vi "RTS Door Opener Server Side.vi"() -> ()   [LabVIEW 2016]
uses:
  <vilib>/Utility/file.llb/Read Delimited Spreadsheet (string).vi
  Type Definitions/RTS Door Open Close Pattern.ctl
  Type Definitions/RTS Door OpenClose Pattern.ctl
  Type Definitions/RTS Door Action.ctl
panel:
  out "Door Open/Close Pattern 4":T1=[{"Door Action"=enum."OPEN", "Timer (Seconds)"=5}, {"Door Action"=enum."CLOSE", "Timer (Seconds)"=5}, {"Door Action"=enum."DELAY", "Timer (Seconds)"=5}, {"Door Action"=enum."REPEAT", "Timer (Seconds)"=0}]
  out "Door Open/Close Pattern 3":T1=[{"Door Action"=enum."OPEN", "Timer (Seconds)"=5}, {"Door Action"=enum."CLOSE", "Timer (Seconds)"=5}, {"Door Action"=enum."DELAY", "Timer (Seconds)"=5}, {"Door Action"=enum."REPEAT", "Timer (Seconds)"=0}]
  out "Door Open/Close Pattern":T1=[{"Door Action"=enum."OPEN", "Timer (Seconds)"=5}, {"Door Action"=enum."CLOSE", "Timer (Seconds)"=5}, {"Door Action"=enum."DELAY", "Timer (Seconds)"=5}, {"Door Action"=enum."REPEAT", "Timer (Seconds)"=0}]
  in  "OK":bool
  out "Elapsed days":i32
  out "End Time":timestamp format="%<%I:%M:%S%3u %p\n%m/%d/%Y>T"
  out "Start Time":timestamp format="%<%I:%M:%S%3u %p\n%m/%d/%Y>T"
  in  "Path":path
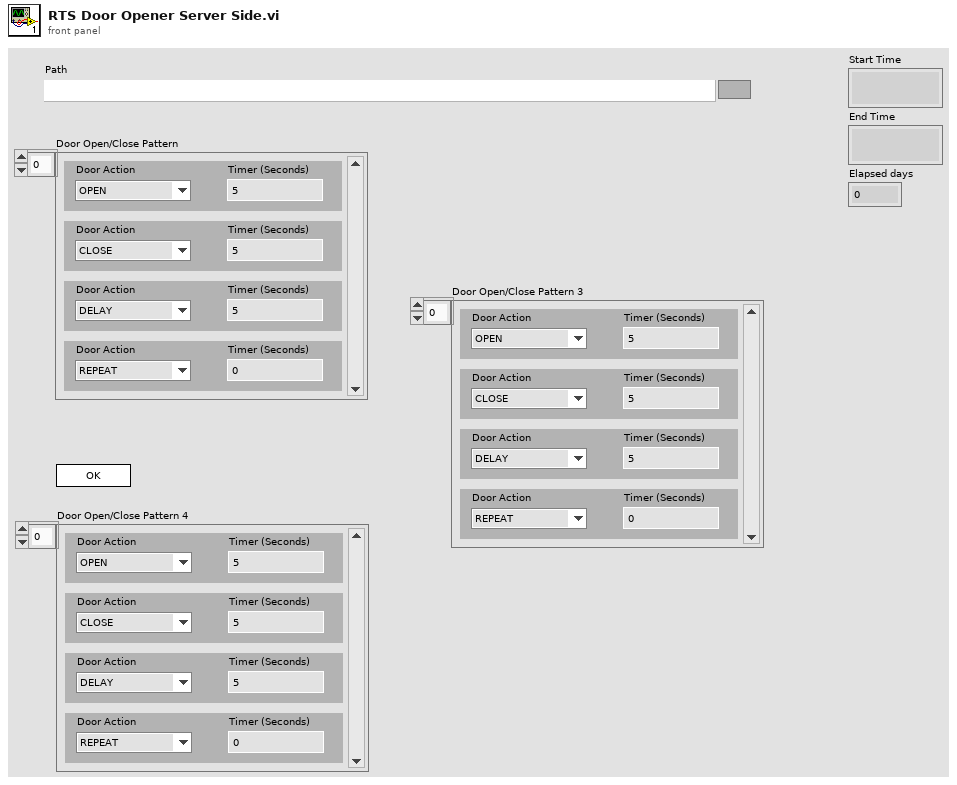
[diagram p1: front panel]
types:
  T1 = typedef "RTS Door OpenClose Pattern.ctl" = T2[]
  T2 = typedef "RTS Door Open Close Pattern.ctl" = cluster{"Door Action":T3, "Timer (Seconds)":u16}
  T3 = typedef "RTS Door Action.ctl" = enum16{"OPEN", "CLOSE", "DELAY", "REPEAT"}
  T4 = enum32{"invalid app kind", "Development System", "Run Time System", "Student Edition", "Embedded LabVIEW", "Evaluation", "Custom"}
  T5 = enum32{"Invalid", "Standard", "Closed", "Hidden", "Minimized", "Maximized"}
  T6 = cluster{"Core":cluster{"Current VI Reference":refnum<vi>, "Close Panel on Exit?":bool}, "Path":path, "Door Open/Close Pattern":T1, "End Time Const ":timestamp, "Start Time Const":timestamp}
  T7 = cluster{"Current VI Reference":refnum<vi>, "Close Panel on Exit?":bool}
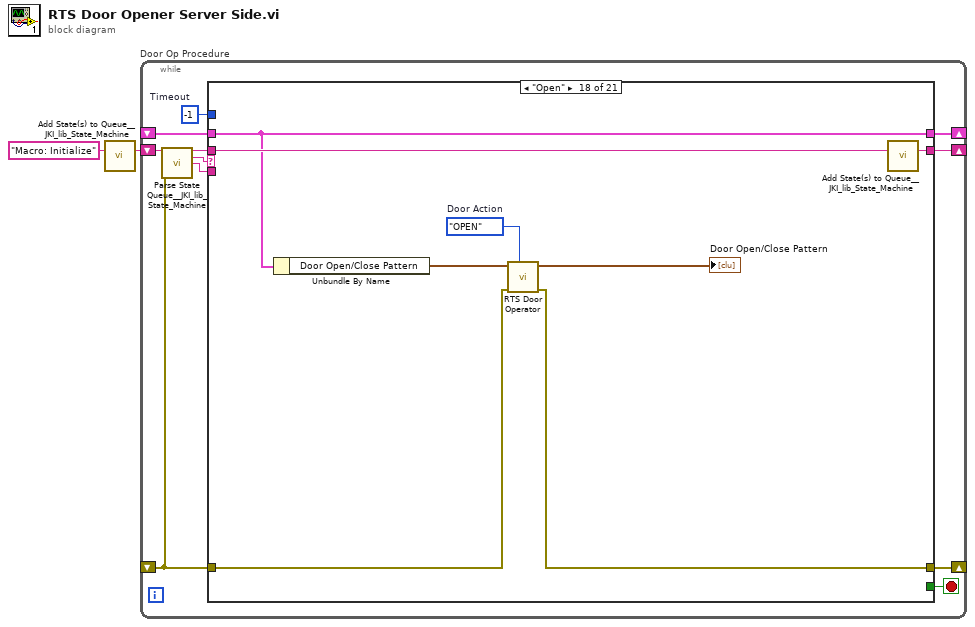
[diagram p0: block diagram]
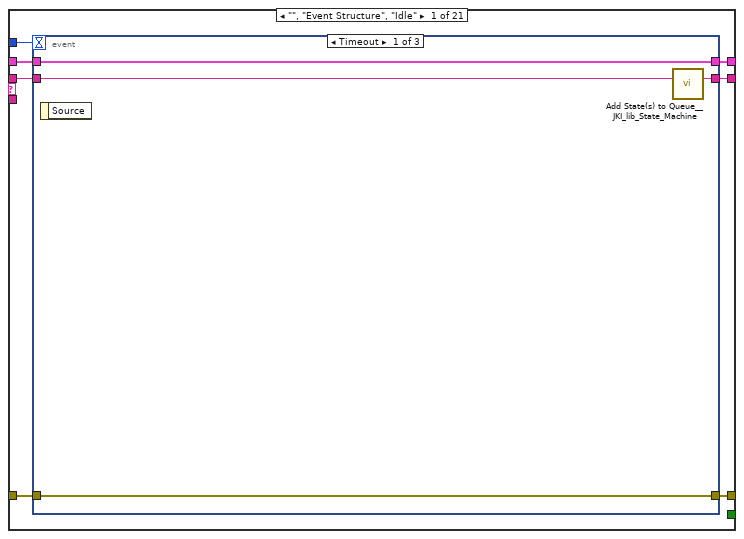
[diagram p2: hidden frame]
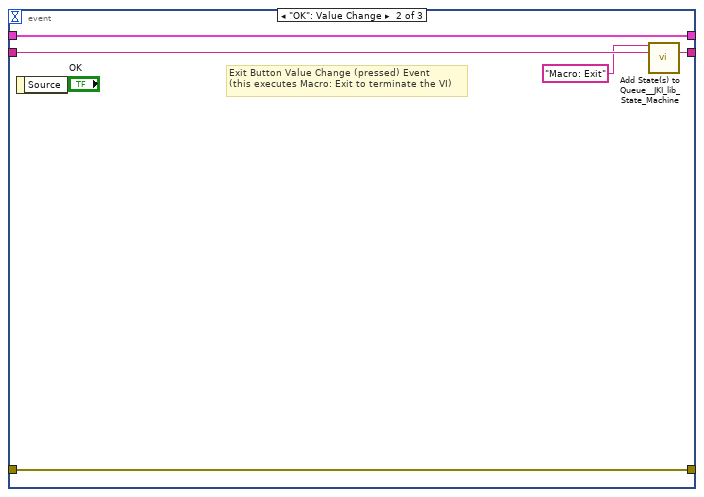
[diagram p3: hidden frame]
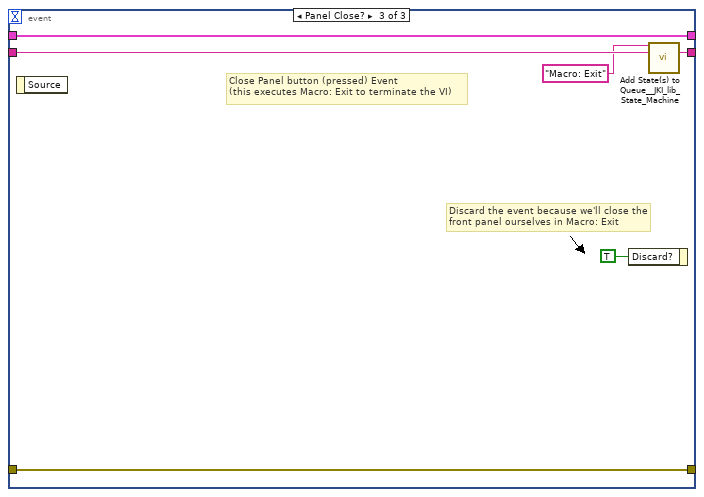
[diagram p4: hidden frame]
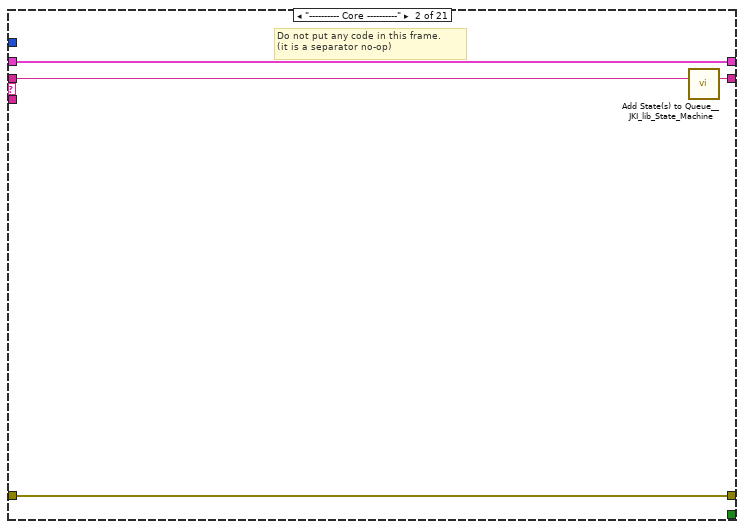
[diagram p5: hidden frame]
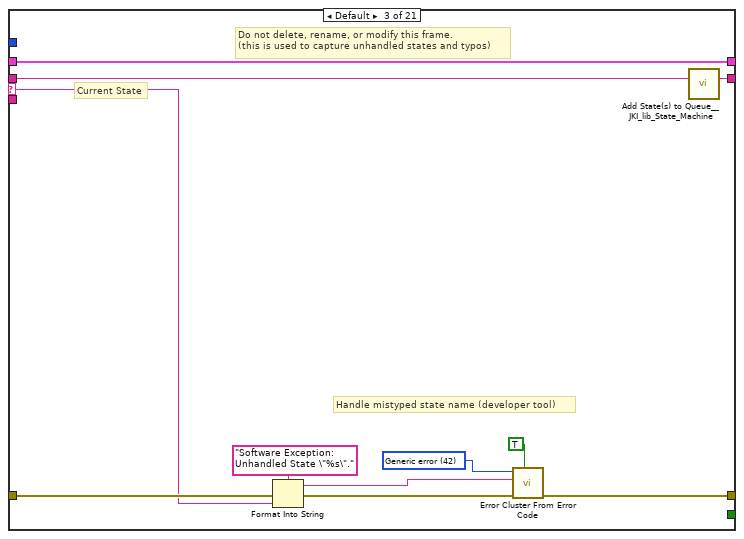
[diagram p6: hidden frame]
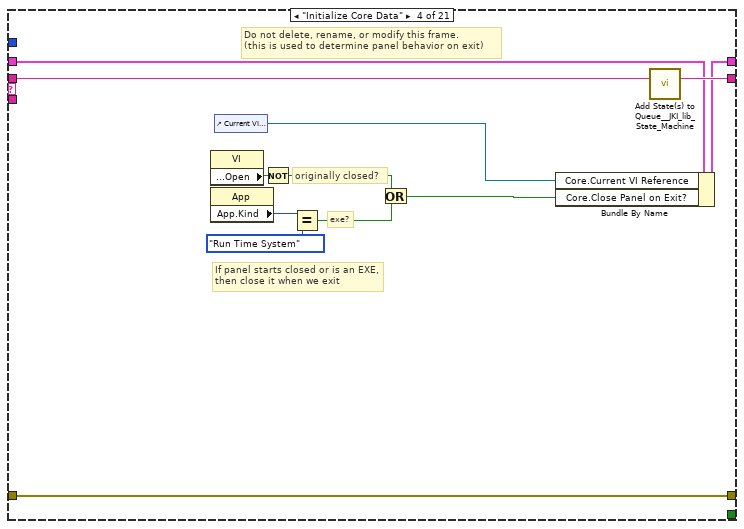
[diagram p7: hidden frame]
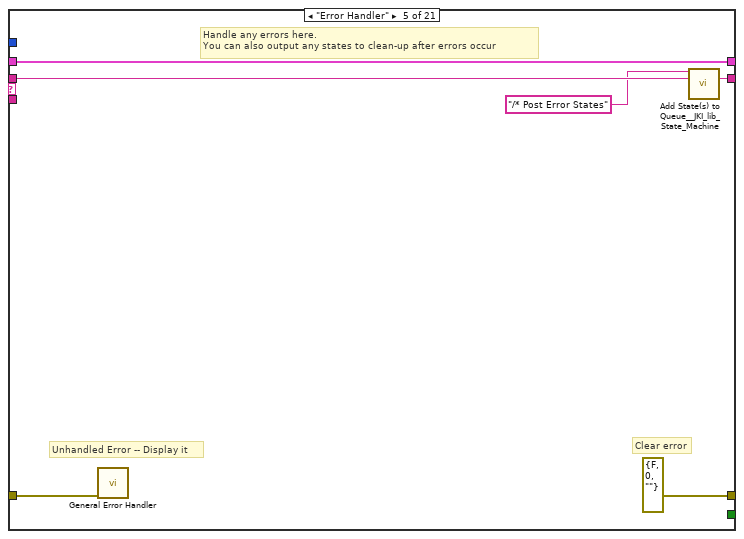
[diagram p8: hidden frame]
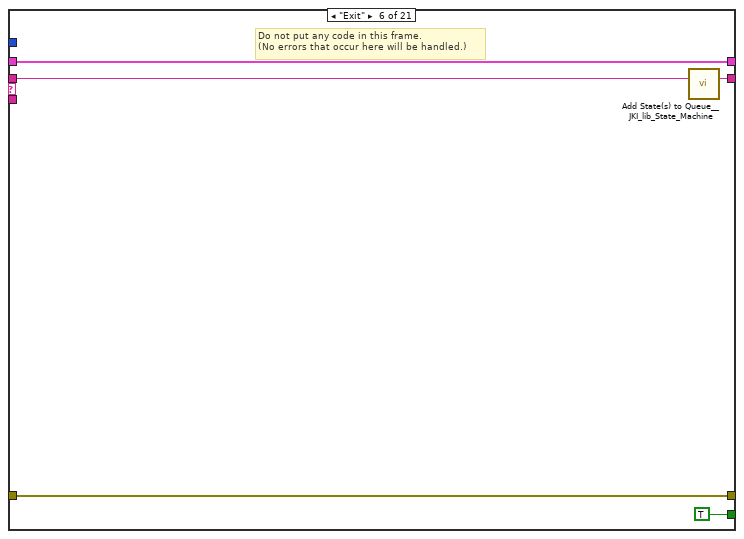
[diagram p9: hidden frame]
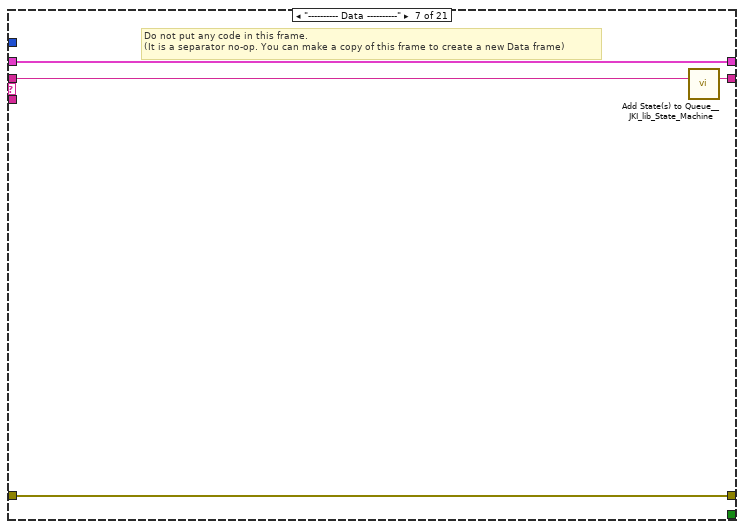
[diagram p10: hidden frame]
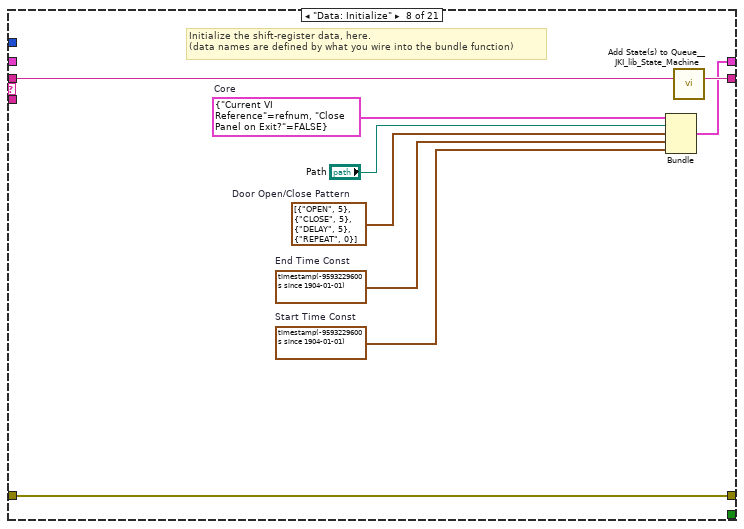
[diagram p11: hidden frame]
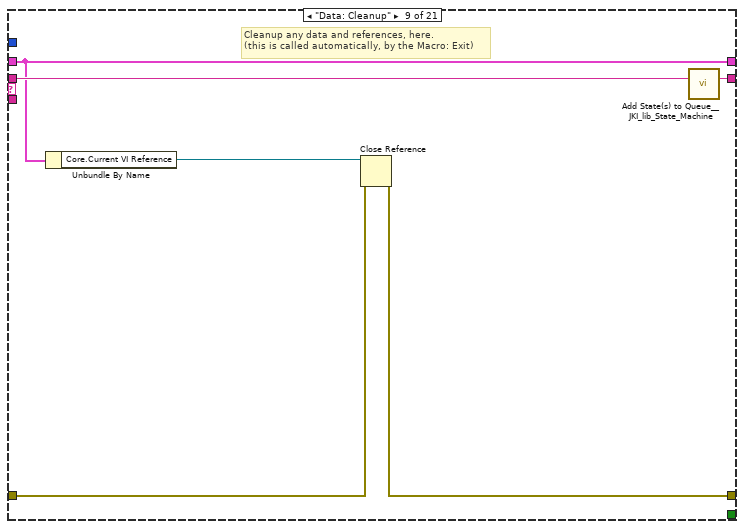
[diagram p12: hidden frame]
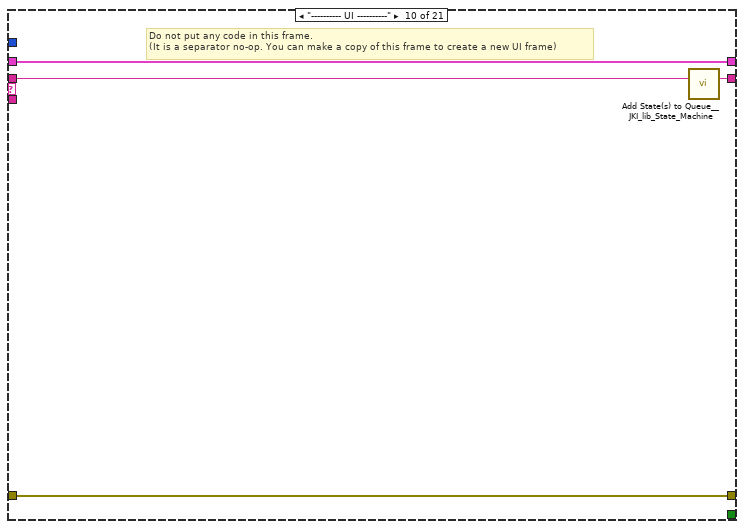
[diagram p13: hidden frame]
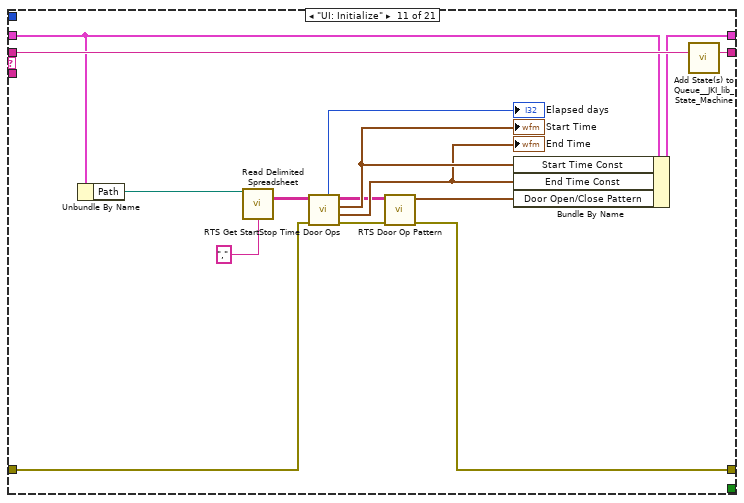
[diagram p14: hidden frame]
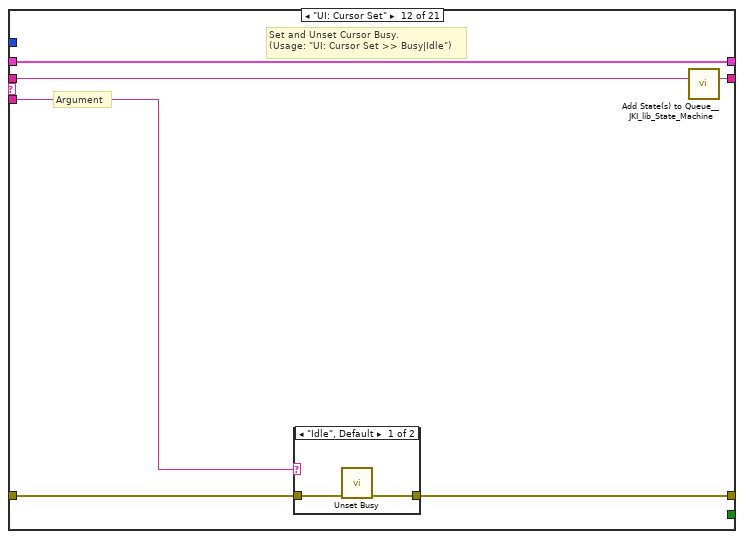
[diagram p15: hidden frame]
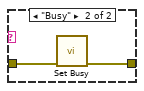
[diagram p16: hidden frame]
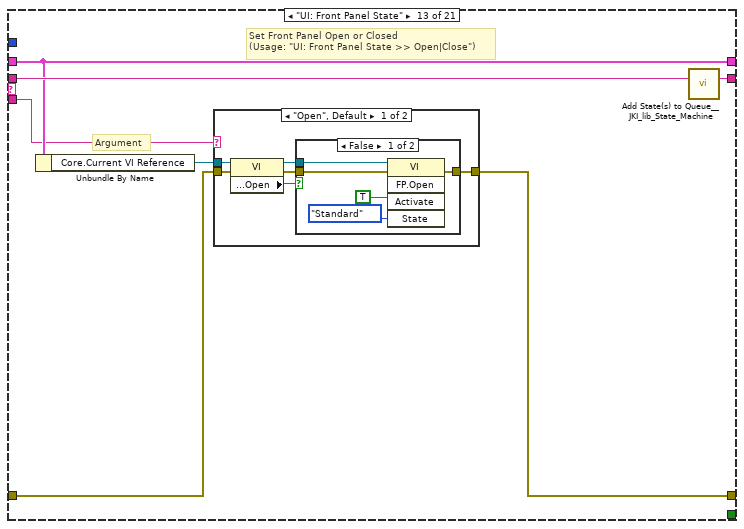
[diagram p17: hidden frame]
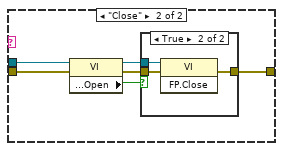
[diagram p19: hidden frame]
diagram:
  n1 = call <vilib>:"Add State(s) to Queue__JKI_lib_State_Machine.vi"("State(s) in (\"\")"="Macro: Initialize") -> ("States Out"=w2:string)  [unwired: 14 in]
  n2 = while "Door Op Procedure" {
    shift-right: [w6] -> _
    shift-left: _ -> [w5]
    shift-right: [w9] -> _
    shift-left: _ -> [w3]
    shift-right: [w8] -> _
    shift-left: w2 -> [w10]
    stop <- w7 stop-if-true
    w4 = -1  # Timeout
    n3 = call <vilib>:"Parse State Queue__JKI_lib_State_Machine.vi"("State Queue"=w10, "Error In (no error)"=w3) -> ("Remaining States"=w12:string, "Current State"=w13:string, "Arguments"=w11:string)  [unwired: 11 in]
    n4 = case shown="\"Open\"" w13 {
      selector: w13 -> [_ _ w40 _ _ _ _ _ _ _ _ _ _ _ _ _ _ _ _ _ _]
      tunnel: w12 -> [w20 w39 w44 w62 w68 w73 w77 w86 w92 w96 w111 w117 w128 w154 w159 w169 w173 w181 w189 w197 w201]
      tunnel: w11 -> [_ _ _ _ _ _ _ _ _ _ _ w112 w122 _ _ _ _ _ _ _ _]
      tunnel: w5 -> [w18 w36 w42 w53 w65 w71 w74 _ w87 w93 w106 w115 w124 w151 w156 w166 w170 w179 w184 w192 w198]
      tunnel: [w17 w37 w46 w59 errorcluster {"status"=FALSE, "code"=0, "source"=""} ("error out") w70 w75 w83 w88 w94 w98 w113 w125 w152 w157 w167 w171 w175 w182 w190 w199] -> w9
      tunnel: w3 -> [w16 w37 w45 w59 w64 w70 w75 w83 w89 w94 w103 w114 w126 w152 w157 w167 w171 w176 w183 w191 w199]
      tunnel: [w19 w38 w43 w61 w67 w72 w76 w85 w91 w95 w110 w116 w127 w153 w158 w168 w172 w180 w188 w196 w200] -> w8
      tunnel: [_ _ _ _ _ TRUE _ _ _ _ _ _ _ _ _ _ _ _ _ _ _] -> w7
      tunnel: [w15 w36 w42 w60 w65 w71 w74 w84 w87 w93 w105 w115 w124 w151 w156 w166 w170 w179 w184 w192 w198] -> w6
      tunnel: w4 -> [w14 _ _ _ _ _ _ _ _ _ _ _ _ _ _ _ _ _ _ _ _]
      frame "", "Event Structure", "Idle" {
        n5 = event shown="[0] Timeout" {
          selector: _ -> [_ _ _]
          dyn-events: _ -> [_ _ _]
          timeout: w14 -> [_ _ _]
          tunnel: w20 -> [w24 w29 w35]
          tunnel: [w23 w28 w34] -> w19
          tunnel: w18 -> [w21 w26 w32]
          tunnel: [w22 w27 w33] -> w17
          tunnel: w16 -> [w22 w27 w33]
          tunnel: [w21 w26 w32] -> w15
          event Timeout {
            n6 = event-data() -> ()  [unwired: 1 in, 1 out]
            n7 = call <vilib>:"Add State(s) to Queue__JKI_lib_State_Machine.vi"("State(s) in (\"\")"=w24) -> ("States Out"=w23:string)  [unwired: 14 in]
          }
          event "OK": Value Change {
            # "Exit Button Value Change (pressed) Event\n(this executes Macro: Exit to terminate the VI)"
            n8 = event-data() -> ()  [unwired: 1 in, 1 out]
            n9 = call <vilib>:"Add State(s) to Queue__JKI_lib_State_Machine.vi"("State(s) in Front (\"\")"="Macro: Exit", "State(s) in (\"\")"=w29) -> ("States Out"=w28:string)  [unwired: 13 in]
          }
          event Panel Close? {
            # "Discard the event because we'll close the front panel ourselves in Macro: Exit"
            # "Close Panel button (pressed) Event\n(this executes Macro: Exit to terminate the VI)"
            n10 = event-data() -> ()  [unwired: 1 in, 1 out]
            n11 = event-data("Discard?"=TRUE) -> ()  [unwired: 1 in, 1 out]
            n12 = call <vilib>:"Add State(s) to Queue__JKI_lib_State_Machine.vi"("State(s) in Front (\"\")"="Macro: Exit", "State(s) in (\"\")"=w35) -> ("States Out"=w34:string)  [unwired: 13 in]
          }
        }
      }
      frame "---------- Core ----------" {
        # "Do not put any code in this frame.\n(it is a separator no-op)"
        n13 = call <vilib>:"Add State(s) to Queue__JKI_lib_State_Machine.vi"("State(s) in (\"\")"=w39) -> ("States Out"=w38:string)  [unwired: 14 in]
      }
      frame Default {
        w49 = 42 items=["No error", "Argument error", "Memory is full", "Out of zone", "End of file", "File already open", "Generic file I/O error", "File not found", "File permission error", "Disk is full", "Duplicate path", "Too many files open", "System feature not enabled", "Resource file not found", "Cannot add resource", "Resource not found", "Image not found", "Image memory error", "Pen does not exist", "Config type invalid", "Config token not found", "Config parse error", "Config memory error", "Bad external code format", "Bad external code offset", "External code not present", "Null window", "Destroy window error", "Null menu", "Print aborted", "Bad print record", "Print driver error", "Windows error during printing", "Memory error during printing", "Print dialog error", "Generic print error", "Invalid device refnum", "Device not found", "Device parameter error", "Device unit error", "Cannot open device", "Device call aborted", "Generic error", "Cancelled by user", "Object ID too low", "Object ID too high", "Object not in heap", "Unknown heap", "Unknown object (invalid DefProc)", "Unknown object (DefProc not in table)", "Message out of range", "Invalid (null) method", "Unknown message", "Manager call not supported", "Bad address", "Network operation in progress", "Network operation timed out", "Connection is busy", "Network attribute not supported", "Network error", "Address in use", "System out of memory", "Connection aborted", "Connection refused", "Not connected", "Already connected", "Connection closed", "Initialization error (interapplication manager)", "Bad occurrence", "Wait on unbound occurrence handler", "Occurrence queue overflow", "Datalog type conflict", "Unused", "Unrecognized type (interapplication manager)", "Memory corrupt", "Failed to make temporary DLL", "Old CIN version", "Drag socket not found", "Failed to load drop-object", "Failed to register OLE object", "Failed to release OLE object", "Format specifier type mismatch", "Unknown format specifier", "Too few format specifiers", "Too many format specifiers", "Scan failed", "Newer CIN version", "Error converting to variant", "Runtime menu error", "Password tampered", "Variant attribute not found", "Incompatible variant data type", "Event data is not available", "Event Store is not present", "Occurrence is not found", "Event Queue is not created", "Event info is not available", "Refnum passed is NULL", "Error retrieving Class GUID", "Error retrieving CoClass GUID", "Error retrieving TypeLib GUID.", "Bad built application magic bytes.", "Specific driver is different from the specific driver associated with the Logical Name.", "There is no session opened to the class driver.", "Max Error", "MAX - Error with config objects", "MAX - Error loading configuration", "MAX - Group not supported"]
        # "Current State"
        # "Do not delete, rename, or modify this frame.\n(this is used to capture unhandled states and typos)"
        # "Handle mistyped state name (developer tool)"
        n14 = Format Into String(format string="Software Exception: Unhandled State \"%s\"." ("message"), error in=w45, w40) -> (resulting string=w48:string, error out=w47:errorcluster)  [unwired: 1 in]
        n15 = call <vilib>:"Error Cluster From Error Code.vi"("show call chain? (False)"=TRUE, "error in (no error)"=w47, "error message (\"\")"=w48, "error code (0)"=w49) -> ("error out"=w46:errorcluster)  [unwired: 5 in]
        n16 = call <vilib>:"Add State(s) to Queue__JKI_lib_State_Machine.vi"("State(s) in (\"\")"=w44) -> ("States Out"=w43:string)  [unwired: 14 in]
      }
      frame "Initialize Core Data" {
        # "Do not delete, rename, or modify this frame.\n(this is used to determine panel behavior on exit)"
        # "originally closed?"
        # "exe?"
        # "If panel starts closed or is an EXE, then close it when we exit"
        n17 = property class="VI"() -> ("Front Panel.Open"=w58:bool)  [unwired: 2 in, 2 out]
        n18 = property class="App"() -> ("App.Kind"=w57:T4)  [unwired: 2 in, 2 out]
        n19 = control-ref of="Current VI Reference"() -> (w51:refnum<vi>)
        n20 = Not(x=w58) -> (.not. x?=w55:bool)
        n21 = Equal?(x=w57, y=T4."Run Time System" ("Application:Kind")) -> (x = y?=w54:bool)
        n22 = Or(x=w55, y=w54) -> (x .or. y?=w52:bool)
        n23 = Bundle By Name(cluster=w53, "Core.Current VI Reference"=w51, "Core.Close Panel on Exit?"=w52) -> (w60:T6)
        n24 = call <vilib>:"Add State(s) to Queue__JKI_lib_State_Machine.vi"("State(s) in (\"\")"=w62) -> ("States Out"=w61:string)  [unwired: 14 in]
      }
      frame "Error Handler" {
        # "Unhandled Error -- Display it"
        # "Handle any errors here.\nYou can also output any states to clean-up after errors occur"
        # "Clear error"
        n25 = call <vilib>:"General Error Handler.vi"("error in (no error)"=w64) -> ()  [unwired: 10 in, 5 out]
        n26 = call <vilib>:"Add State(s) to Queue__JKI_lib_State_Machine.vi"("State(s) in Front (\"\")"="/* Post Error States", "State(s) in (\"\")"=w68) -> ("States Out"=w67:string)  [unwired: 13 in]
      }
      frame "Exit" {
        # "Do not put any code in this frame.\n(No errors that occur here will be handled.)"
        n27 = call <vilib>:"Add State(s) to Queue__JKI_lib_State_Machine.vi"("State(s) in (\"\")"=w73) -> ("States Out"=w72:string)  [unwired: 14 in]
      }
      frame "---------- Data ----------" {
        # "Do not put any code in this frame.\n(It is a separator no-op. You can make a copy of this frame to create a new Data frame)"
        n28 = call <vilib>:"Add State(s) to Queue__JKI_lib_State_Machine.vi"("State(s) in (\"\")"=w77) -> ("States Out"=w76:string)  [unwired: 14 in]
      }
      frame "Data: Initialize" {
        w80 = T1 [{"Door Action"=enum."OPEN", "Timer (Seconds)"=5}, {"Door Action"=enum."CLOSE", "Timer (Seconds)"=5}, {"Door Action"=enum."DELAY", "Timer (Seconds)"=5}, {"Door Action"=enum."REPEAT", "Timer (Seconds)"=0}]  # Door Open/Close Pattern
        w78 = timestamp(-9593229600 s since 1904-01-01)  # Start Time Const
        w79 = timestamp(-9593229600 s since 1904-01-01)  # End Time Const
        w82 = T7 {"Current VI Reference"=refnum, "Close Panel on Exit?"=FALSE}  # Core
        # "Initialize the shift-register data, here.\n(data names are defined by what you wire into the bundle function)"
        n29 = Bundle("Core"=w82, "Path"="Path", "Door Open/Close Pattern"=w80, "End Time Const"=w79, "Start Time Const"=w78) -> (w84:T6)  [unwired: 1 in]
        n30 = call <vilib>:"Add State(s) to Queue__JKI_lib_State_Machine.vi"("State(s) in (\"\")"=w86) -> ("States Out"=w85:string)  [unwired: 14 in]
      }
      frame "Data: Cleanup" {
        # "Cleanup any data and references, here.\n(this is called automatically, by the Macro: Exit)"
        n31 = Unbundle By Name(w87) -> ("Core.Current VI Reference"=w90:refnum<vi>)
        n32 = Close Reference(reference=w90, error in (no error)=w89) -> (error out=w88:errorcluster)
        n33 = call <vilib>:"Add State(s) to Queue__JKI_lib_State_Machine.vi"("State(s) in (\"\")"=w92) -> ("States Out"=w91:string)  [unwired: 14 in]
      }
      frame "---------- UI ----------" {
        # "Do not put any code in this frame.\n(It is a separator no-op. You can make a copy of this frame to create a new UI frame)"
        n34 = call <vilib>:"Add State(s) to Queue__JKI_lib_State_Machine.vi"("State(s) in (\"\")"=w96) -> ("States Out"=w95:string)  [unwired: 14 in]
      }
      frame "UI: Initialize" {
        n35 = Unbundle By Name(w106) -> ("Path"=w107:path)
        n36 = call-poly <vilib>:"Read Delimited Spreadsheet.vi"("file path (dialog if empty)"=w107, "delimiter (\\t)"="," ("delimiter (\\t)")) -> ("all rows"=w109:string[][])  [unwired: 8 in, 5 out]
        n37 = call "RTS Get StartStop Time Door Ops.vi"("Error In"=w103, "Door Op Data Input"=w109) -> ("Error Out"=w99:errorcluster, "End Time"=w101:timestamp, "Start Time"=w102:timestamp, "Door Op Data Output"=w100:string[][], "Elapsed days"=→"Elapsed days":i32)  [unwired: 5 in]
        "Start Time" <- w102
        "End Time" <- w101
        n38 = call "RTS Door Op Pattern.vi"("Error In"=w99, "Door Op Data Input"=w100) -> ("Error Out"=w98:errorcluster, "Door Op Pattern"=w97:T2[])  [unwired: 8 in]
        n39 = Bundle By Name(cluster=w106, "Start Time Const"=w102, "End Time Const"=w101, "Door Open/Close Pattern"=w97) -> (w105:T6)
        n40 = call <vilib>:"Add State(s) to Queue__JKI_lib_State_Machine.vi"("State(s) in (\"\")"=w111) -> ("States Out"=w110:string)  [unwired: 14 in]
      }
      frame "UI: Cursor Set" {
        # "Argument"
        # "Set and Unset Cursor Busy.\n(Usage: \"UI: Cursor Set >> Busy|Idle\")"
        n41 = case shown="\"Idle\", Default" w112 {
          tunnel: w114 -> [w119 w121]
          tunnel: [w118 w120] -> w113
          frame "Idle", Default {
            n42 = call <vilib>:"Unset Busy.vi"("error in (no error)"=w119) -> ("error out"=w118:errorcluster)  [unwired: 10 in]
          }
          frame "Busy" {
            n43 = call <vilib>:"Set Busy.vi"("error in (no error)"=w121) -> ("error out"=w120:errorcluster)  [unwired: 9 in, 1 out]
          }
        }
        n44 = call <vilib>:"Add State(s) to Queue__JKI_lib_State_Machine.vi"("State(s) in (\"\")"=w117) -> ("States Out"=w116:string)  [unwired: 14 in]
      }
      frame "UI: Front Panel State" {
        # "Argument"
        # "Set Front Panel Open or Closed\n(Usage: \"UI: Front Panel State >> Open|Close\")"
        n45 = Unbundle By Name(w124) -> ("Core.Current VI Reference"=w123:refnum<vi>)
        n46 = case shown="\"Open\", Default" w122 {
          tunnel: w126 -> [w132 w145]
          tunnel: [w134 w146] -> w125
          tunnel: w123 -> [w133 w143]
          frame "Open", Default {
            n47 = property class="VI"(reference=w133, error in=w132) -> (reference out=w130:refnum<vi>, error out=w131:errorcluster, "Front Panel.Open"=w129:bool)
            n48 = case shown="False" w129 {
              tunnel: [w137 w140] -> w134
              tunnel: w131 -> [w136 w140]
              tunnel: w130 -> [w135 _]
              frame False {
                n49 = invoke class="VI" method="FP.Open"(reference=w135, error in=w136, "Activate"=TRUE, "State"=T5."Standard") -> (error out=w137:errorcluster)  [unwired: 1 in, 4 out]
              }
              frame True {
              }
            }
          }
          frame "Close" {
            n50 = property class="VI"(reference=w143, error in=w145) -> (reference out=w142:refnum<vi>, error out=w144:errorcluster, "Front Panel.Open"=w141:bool)
            n51 = case shown="True" w141 {
              tunnel: [w147 w150] -> w146
              tunnel: w144 -> [w147 w149]
              tunnel: w142 -> [_ w148]
              frame False {
              }
              frame True {
                n52 = invoke class="VI" method="FP.Close"(reference=w148, error in=w149) -> (error out=w150:errorcluster)  [unwired: 1 in, 2 out]
              }
            }
          }
        }
        n53 = call <vilib>:"Add State(s) to Queue__JKI_lib_State_Machine.vi"("State(s) in (\"\")"=w128) -> ("States Out"=w127:string)  [unwired: 14 in]
      }
      frame "---------- Macro ----------" {
        # "Do not put any code in this frame.\n(It is a separator no-op. You can make a copy of this frame to create a new Macro frame)"
        n54 = call <vilib>:"Add State(s) to Queue__JKI_lib_State_Machine.vi"("State(s) in (\"\")"=w154) -> ("States Out"=w153:string)  [unwired: 14 in]
      }
      frame "Macro: Initialize" {
        w155 = "Data: Initialize\nInitialize Core Data\nUI: Initialize\nUI: Front Panel State >> Open"  # Data: Initialize Initialize Core Data UI: Initialize UI: Front Panel State >> Open
        # "Initialization Macro\n(This is called once, when the VI starts)"
        n55 = call <vilib>:"Add State(s) to Queue__JKI_lib_State_Machine.vi"("State(s) in Front (\"\")"=w155, "State(s) in (\"\")"=w159) -> ("States Out"=w158:string)  [unwired: 13 in]
      }
      frame "Macro: Exit" {
        # "Exit Macro\n(This is called once, when the VI exits)"
        n56 = Unbundle By Name(w166) -> ("Core.Close Panel on Exit?"=w165:bool)
        n57 = Select(t="UI: Front Panel State >> Close", s=w165, f="") -> (s? t:f=w162:string)
        n58 = call <vilib>:"Add State(s) to Queue__JKI_lib_State_Machine.vi"("State(s) in (\"\")"=w162, "State(s) at Back (\"\")"="Data: Cleanup\nExit") -> ("States Out"=w160:string)  [unwired: 13 in]
        n59 = call <vilib>:"Add State(s) to Queue__JKI_lib_State_Machine.vi"("State(s) in Front (\"\")"=w160, "State(s) in (\"\")"=w169) -> ("States Out"=w168:string)  [unwired: 13 in]
      }
      frame "---------- New Category ----------" {
        # "Template Separator\n(You can make a copy of, or modify, this frame)"
        n60 = call <vilib>:"Add State(s) to Queue__JKI_lib_State_Machine.vi"("State(s) in (\"\")"=w173) -> ("States Out"=w172:string)  [unwired: 14 in]
      }
      frame "Open" {
        w174 = RTS_Door_Action."OPEN"  # Door Action
        n61 = Unbundle By Name(w179) -> ("Door Open/Close Pattern"=w178:T1)
        n62 = call "RTS Door Operator.vi"("Door Action"=w174, "Error In"=w176, "Door Open/Close Pattern in"=w178) -> ("Error Out"=w175:errorcluster, "Door Open/Close Pattern out"=→"Door Open/Close Pattern":T1)  [unwired: 7 in]
        n63 = call <vilib>:"Add State(s) to Queue__JKI_lib_State_Machine.vi"("State(s) in (\"\")"=w181) -> ("States Out"=w180:string)  [unwired: 14 in]
      }
      frame "Close" {
        w185 = RTS_Door_Action."CLOSE"  # Door Action
        n64 = Unbundle By Name(w184) -> ("Door Open/Close Pattern"=w187:T1)
        n65 = call "RTS Door Operator.vi"("Door Action"=w185, "Error In"=w183, "Door Open/Close Pattern in"=w187) -> ("Error Out"=w182:errorcluster, "Door Open/Close Pattern out"=→"Door Open/Close Pattern 3":T1)  [unwired: 7 in]
        n66 = call <vilib>:"Add State(s) to Queue__JKI_lib_State_Machine.vi"("State(s) in (\"\")"=w189) -> ("States Out"=w188:string)  [unwired: 14 in]
      }
      frame "Delay" {
        w193 = RTS_Door_Action."DELAY"  # Door Action
        n67 = Unbundle By Name(w192) -> ("Door Open/Close Pattern"=w195:T1)
        n68 = call "RTS Door Operator.vi"("Door Action"=w193, "Error In"=w191, "Door Open/Close Pattern in"=w195) -> ("Error Out"=w190:errorcluster, "Door Open/Close Pattern out"=→"Door Open/Close Pattern 4":T1)  [unwired: 7 in]
        n69 = call <vilib>:"Add State(s) to Queue__JKI_lib_State_Machine.vi"("State(s) in (\"\")"=w197) -> ("States Out"=w196:string)  [unwired: 14 in]
      }
      frame "Repeat" {
        (unwired) RTS_Door_Action."REPEAT"  # Door Action
        n70 = call <vilib>:"Add State(s) to Queue__JKI_lib_State_Machine.vi"("State(s) in (\"\")"=w201) -> ("States Out"=w200:string)  [unwired: 14 in]
      }
    }
  }
